vi "Set Property.vi"(10 "Ctl Ref":refnum<vi>, 11 "ValueUIP In":refnum<class "ValueUIP.lvclass">) -> (0 "Error Out":errorcluster, 3 "ValueUIP Out":refnum<class "ValueUIP.lvclass">)   [LabVIEW 2020, in "UIM.lvlib" / "ValueUIP.lvclass"]
doc: "Overwrite this abstract method to implement child behavior for applying UIP private data into the VI Server Control property."
uses:
  ValueUIP.lvclass
  ValueUIP.lvclass/ValueUIP.ctl
  <vilib>/Utility/Data Type/NI_Data Type.lvlib
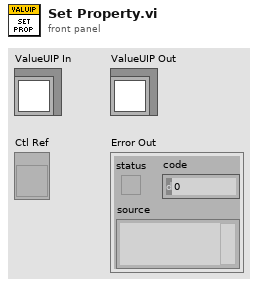
[diagram p1: front panel]
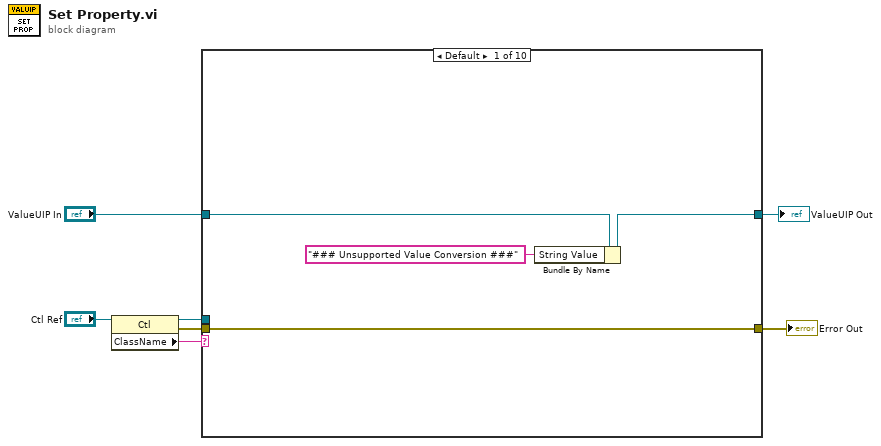
[diagram p0: block diagram]
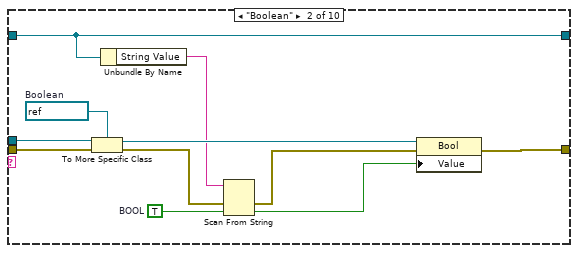
[diagram p2: hidden frame]
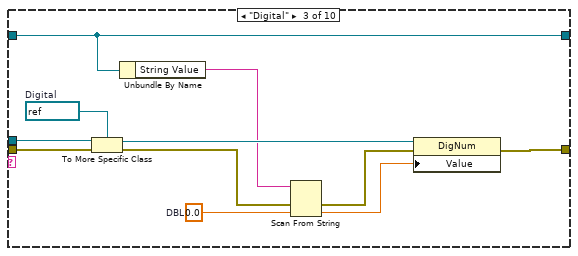
[diagram p3: hidden frame]
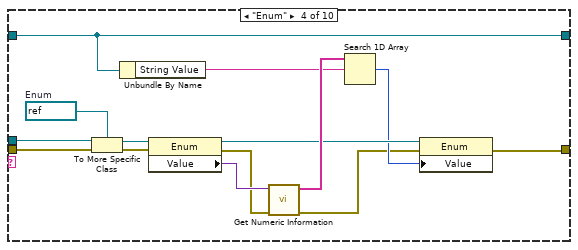
[diagram p4: hidden frame]
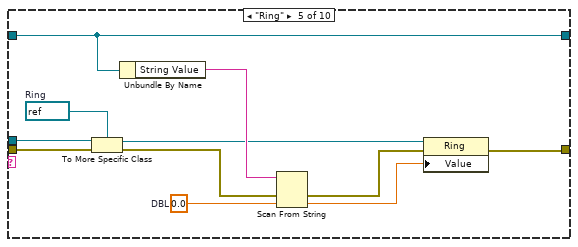
[diagram p5: hidden frame]
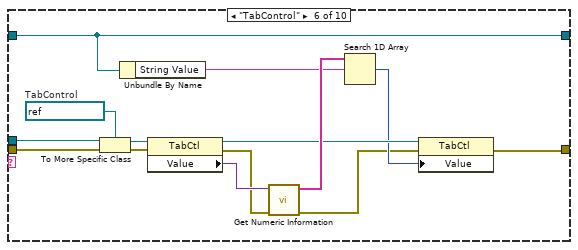
[diagram p6: hidden frame]
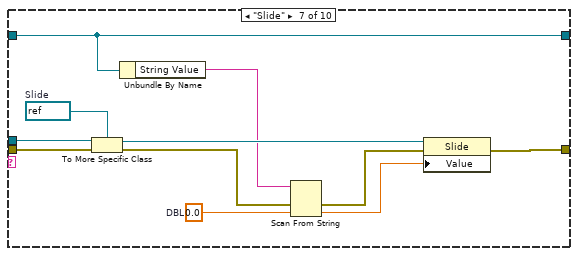
[diagram p7: hidden frame]
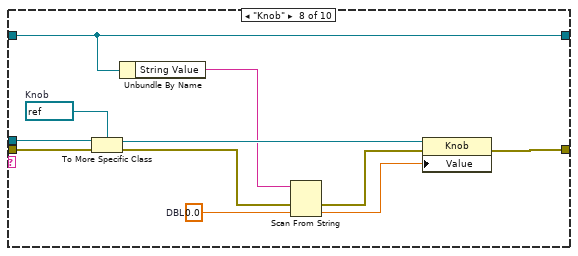
[diagram p8: hidden frame]
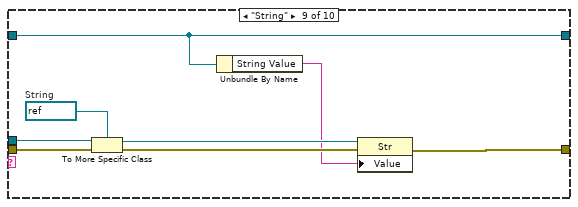
[diagram p9: hidden frame]
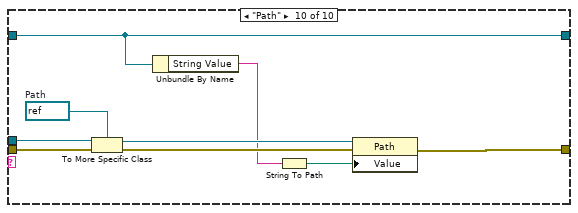
[diagram p10: hidden frame]
diagram:
  n1 = property class="Ctl"(reference="Ctl Ref") -> (reference out=w6:refnum<vi>, error out=w5:errorcluster, "ClassName"=w7:string)  [unwired: 1 in]
  n2 = case shown="Default" w7 {
    tunnel: w6 -> [_ w22 w33 w47 w58 w72 w83 w94 w102 w111]
    tunnel: w5 -> [w11 w21 w32 w46 w57 w71 w82 w93 w101 w110]
    tunnel: "ValueUIP In" -> [w10 w18 w29 w43 w55 w68 w79 w90 w96 w105]
    tunnel: [w9 w18 w29 w43 w55 w68 w79 w90 w96 w105] -> w3
    tunnel: [w11 w13 w28 w34 w54 w59 w78 w89 w97 w106] -> w4
    frame Default {
      n3 = Bundle By Name(cluster=w10, "String Value"="### Unsupported Value Conversion ###") -> (w9:refnum<class "ValueUIP.lvclass">)
    }
    frame "Boolean" {
      w14 = TRUE  # BOOL
      w20 = refnum<vi> refnum  # Boolean
      n4 = To More Specific Class(target class=w20, reference=w22, error in=w21) -> (specific class reference=w19:refnum<vi>, error out=w17:errorcluster)
      n5 = Unbundle By Name(w18) -> ("String Value"=w15:string)
      n6 = Scan From String(input string=w15, error in=w17, default 1=w14) -> (error out=w16:errorcluster, output 1=w12:bool)  [unwired: 2 in, 2 out]
      n7 = property class="Bool"(reference=w19, error in=w16, "Value"=w12) -> (error out=w13:errorcluster)  [unwired: 1 out]
    }
    frame "Digital" {
      w24 = 0.0  # DBL
      w31 = refnum<vi> refnum  # Digital
      n8 = To More Specific Class(target class=w31, reference=w33, error in=w32) -> (specific class reference=w30:refnum<vi>, error out=w27:errorcluster)
      n9 = Unbundle By Name(w29) -> ("String Value"=w23:string)
      n10 = Scan From String(input string=w23, error in=w27, default 1=w24) -> (error out=w26:errorcluster, output 1=w25:dbl)  [unwired: 2 in, 2 out]
      n11 = property class="DigNum"(reference=w30, error in=w26, "Value"=w25) -> (error out=w28:errorcluster)  [unwired: 1 out]
    }
    frame "Enum" {
      w45 = refnum<vi> refnum  # Enum
      n12 = To More Specific Class(target class=w45, reference=w47, error in=w46) -> (specific class reference=w44:refnum<vi>, error out=w42:errorcluster)
      n13 = Unbundle By Name(w43) -> ("String Value"=w38:string)
      n14 = property class="Enum"(reference=w44, error in=w42) -> (reference out=w37:refnum<vi>, error out=w40:errorcluster, "Value"=w41:variant)
      n15 = call <vilib>:"Get Numeric Information.vi"("error in (no error)"=w40, "variant"=w41) -> ("error out"=w35:errorcluster, "enum names"=w39:string[])  [unwired: 6 in, 2 out]
      n16 = Search 1D Array(1D array=w39, element=w38) -> (index of element=w36:i32)  [unwired: 1 in]
      n17 = property class="Enum"(reference=w37, error in=w35, "Value"=w36) -> (error out=w34:errorcluster)  [unwired: 1 out]
    }
    frame "Ring" {
      w49 = 0.0  # DBL
      w56 = refnum<vi> refnum  # Ring
      n18 = To More Specific Class(target class=w56, reference=w58, error in=w57) -> (specific class reference=w51:refnum<vi>, error out=w52:errorcluster)
      n19 = Unbundle By Name(w55) -> ("String Value"=w53:string)
      n20 = Scan From String(input string=w53, error in=w52, default 1=w49) -> (error out=w48:errorcluster, output 1=w50:dbl)  [unwired: 2 in, 2 out]
      n21 = property class="Ring"(reference=w51, error in=w48, "Value"=w50) -> (error out=w54:errorcluster)  [unwired: 1 out]
    }
    frame "TabControl" {
      w70 = refnum<vi> refnum  # TabControl
      n22 = To More Specific Class(target class=w70, reference=w72, error in=w71) -> (specific class reference=w69:refnum<vi>, error out=w67:errorcluster)
      n23 = Unbundle By Name(w68) -> ("String Value"=w63:string)
      n24 = property class="TabCtl"(reference=w69, error in=w67) -> (reference out=w62:refnum<vi>, error out=w65:errorcluster, "Value"=w66:variant)
      n25 = call <vilib>:"Get Numeric Information.vi"("error in (no error)"=w65, "variant"=w66) -> ("error out"=w60:errorcluster, "enum names"=w64:string[])  [unwired: 6 in, 2 out]
      n26 = Search 1D Array(1D array=w64, element=w63) -> (index of element=w61:i32)  [unwired: 1 in]
      n27 = property class="TabCtl"(reference=w62, error in=w60, "Value"=w61) -> (error out=w59:errorcluster)  [unwired: 1 out]
    }
    frame "Slide" {
      w74 = 0.0  # DBL
      w81 = refnum<vi> refnum  # Slide
      n28 = To More Specific Class(target class=w81, reference=w83, error in=w82) -> (specific class reference=w80:refnum<vi>, error out=w77:errorcluster)
      n29 = Unbundle By Name(w79) -> ("String Value"=w73:string)
      n30 = Scan From String(input string=w73, error in=w77, default 1=w74) -> (error out=w76:errorcluster, output 1=w75:dbl)  [unwired: 2 in, 2 out]
      n31 = property class="Slide"(reference=w80, error in=w76, "Value"=w75) -> (error out=w78:errorcluster)  [unwired: 1 out]
    }
    frame "Knob" {
      w85 = 0.0  # DBL
      w92 = refnum<vi> refnum  # Knob
      n32 = To More Specific Class(target class=w92, reference=w94, error in=w93) -> (specific class reference=w91:refnum<vi>, error out=w88:errorcluster)
      n33 = Unbundle By Name(w90) -> ("String Value"=w84:string)
      n34 = Scan From String(input string=w84, error in=w88, default 1=w85) -> (error out=w87:errorcluster, output 1=w86:dbl)  [unwired: 2 in, 2 out]
      n35 = property class="Knob"(reference=w91, error in=w87, "Value"=w86) -> (error out=w89:errorcluster)  [unwired: 1 out]
    }
    frame "String" {
      w100 = refnum<vi> refnum  # String
      n36 = To More Specific Class(target class=w100, reference=w102, error in=w101) -> (specific class reference=w99:refnum<vi>, error out=w98:errorcluster)
      n37 = Unbundle By Name(w96) -> ("String Value"=w95:string)
      n38 = property class="Str"(reference=w99, error in=w98, "Value"=w95) -> (error out=w97:errorcluster)  [unwired: 1 out]
    }
    frame "Path" {
      w109 = refnum<vi> refnum  # Path
      n39 = To More Specific Class(target class=w109, reference=w111, error in=w110) -> (specific class reference=w108:refnum<vi>, error out=w107:errorcluster)
      n40 = Unbundle By Name(w105) -> ("String Value"=w104:string)
      n41 = String To Path(string=w104) -> (path=w103:path)
      n42 = property class="Path"(reference=w108, error in=w107, "Value"=w103) -> (error out=w106:errorcluster)  [unwired: 1 out]
    }
  }
  "Error Out" <- w4
  "ValueUIP Out" <- w3
